vi "msgBandwigthOverload (SubVI).vi"(11 "Mbit/s":string) -> ()   [LabVIEW 2017]
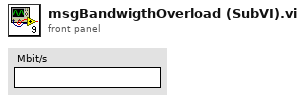
[diagram p1: front panel]
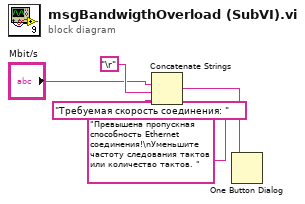
[diagram p0: block diagram]
diagram:
  n1 = Concatenate Strings("Требуемая скорость соединения: " ("string"), "Mbit/s", "\r", "Превышена пропускная способность Ethernet соединения!\nУменьшите частоту следования тактов или количество тактов. " ("message")) -> (w5:string)
  n2 = One Button Dialog(message=w5) -> ()  [unwired: 1 in, 1 out]
